vi "lua_pcall.vi"(7 "msgh":i32, 8 "error in (no error)":errorcluster, 9 "nresults":i32, 10 "nargs":i32, 11 "lua_state_p":u64) -> (0 "error out":errorcluster, 3 "lua_state_p out":u64)   [LabVIEW 2020, in "lua.dll.lvlib"]
uses:
  lua.dll.lvlib
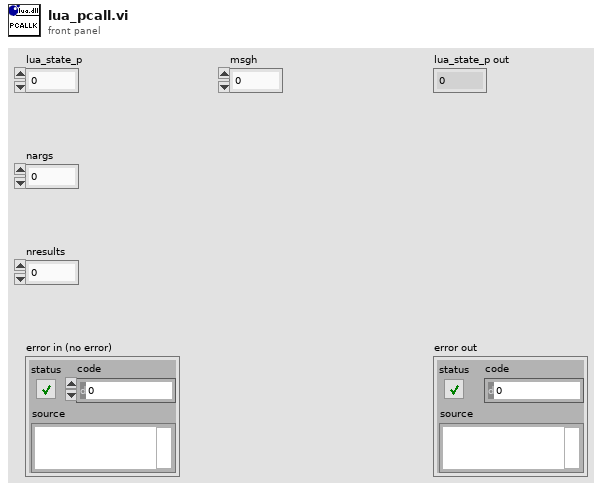
[diagram p1: front panel]
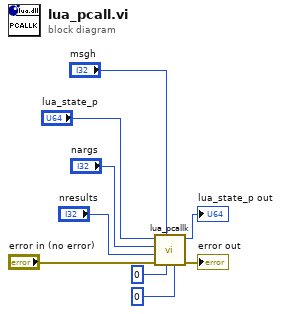
[diagram p0: block diagram]
diagram:
  n1 = call "lua_pcallk.vi"("k"=u64 0, "ctx"=u64 0, "msgh"="msgh", "error in (no error)"="error in (no error)", "nresults"="nresults", "nargs"="nargs", "lua_state_p"="lua_state_p") -> ("error out"=→"error out":errorcluster, "lua_state_p out"=→"lua_state_p out":u64)  [unwired: 3 in]
